vi "FollowPath.vi"(1 "Parameter String":string, 2 "Reinit":bool) -> (0 "Increment":bool)   [LabVIEW 2019]
uses:
  sensors.vi
  dsinstructions.vi
panel:
  out "Azimuth Goal Angle":dbl(knob) scale=180.0..-180.0
  out "FF Contribution":dbl
  out "Distance PID Tracking":cluster{"Goal Wheel Position":dbl, dbl}(graph)={"Goal Wheel Position"=0.0, -90.17571233858979}
  out "Distance Contribution Tracking":cluster{dbl, dbl, dbl}(graph)
  in  "N-Int Distance":i32=5 caption="N-Int"
  in  "N-Diff Distance":i32=10 caption="N-Diff"
  in  "Kd Distance":dbl=0.005
  in  "Ki Distance":dbl=0.2
  in  "Kp Distance":dbl=0.01
  out "Robot Position":cluster{dbl[], dbl[]}[](graph)
  in  "Plot":bool
  in  "N-Int Orientation":i32=10 caption="N-Int"
  in  "N-Diff Orientation":i32=10 caption="N-Diff"
  in  "Kd Orientation":dbl=0.0005
  in  "Ki Orientation":dbl
  in  "Kp Orientation":dbl=0.003
  out "Orientation PID Tracking":cluster{"Goal Wheel Position":dbl, dbl}(graph)={"Goal Wheel Position"=0.0, -90.17571233858979}
  out "Orientation Contribution Tracking":cluster{dbl, dbl, dbl}(graph)
  in  "Look-Ahead Time (s)":dbl=0.25
  in  "Search Window (s)":dbl=2.0
  # "Orientation Control"
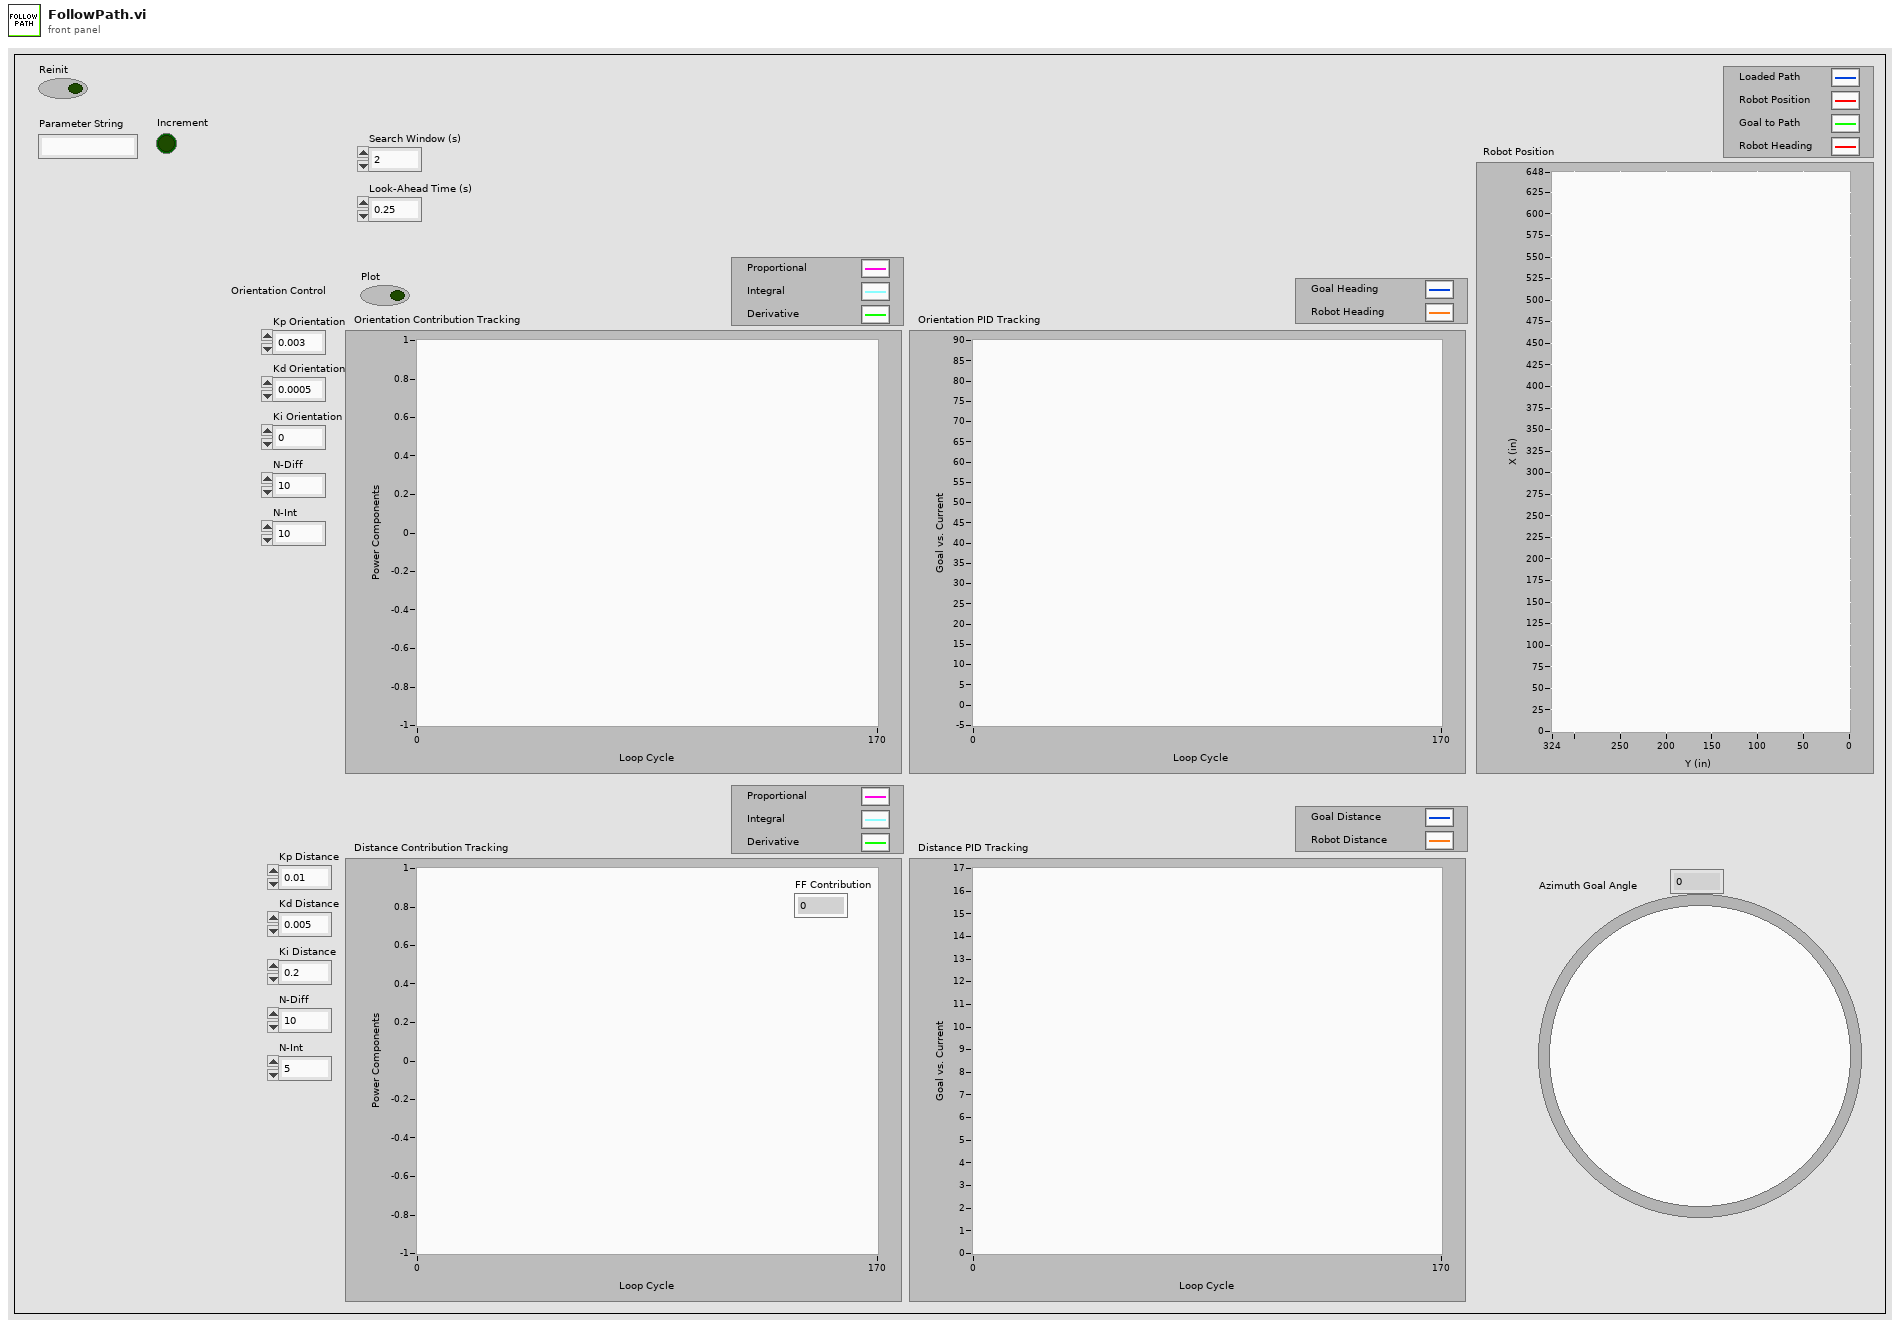
[diagram p1: front panel]
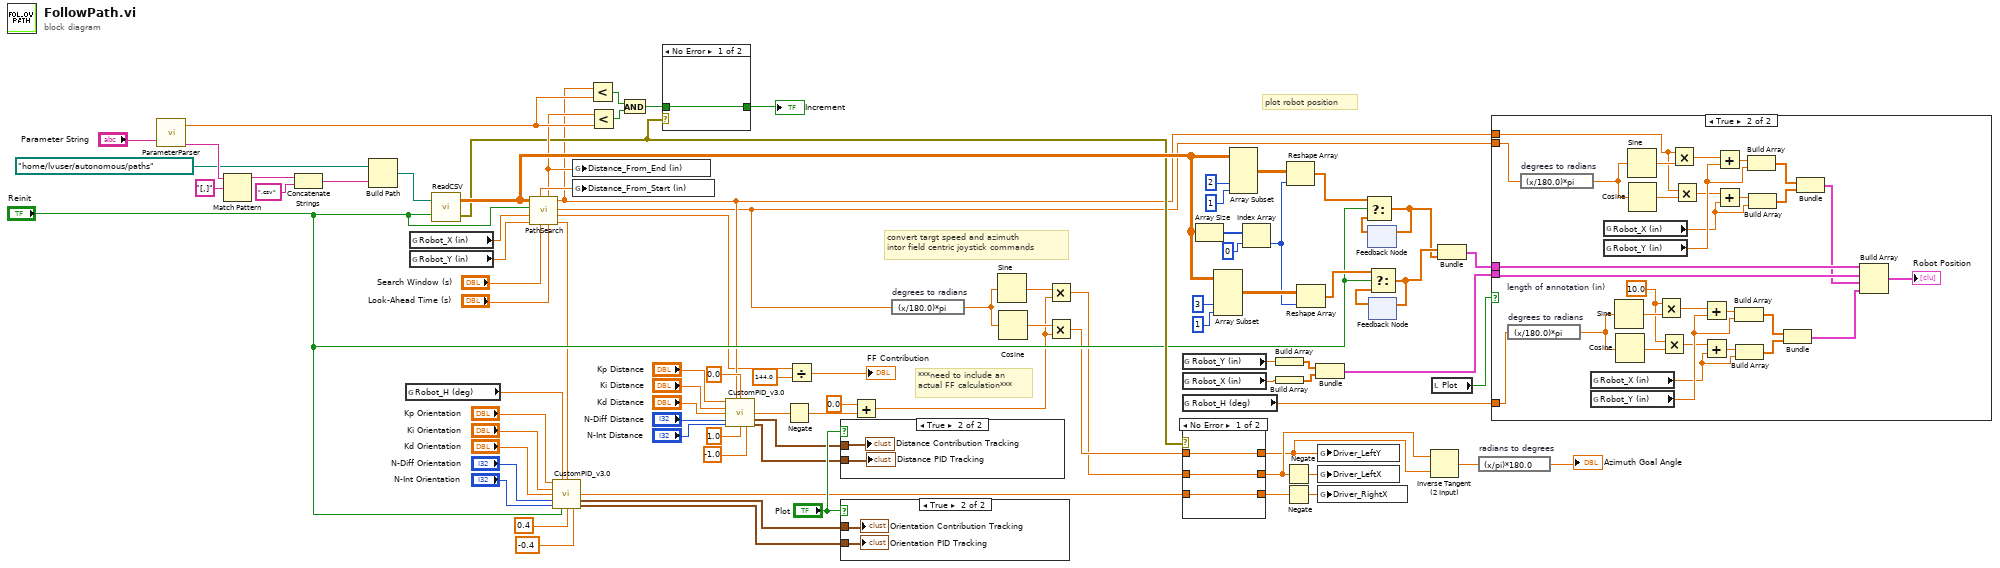
[diagram p0: block diagram]
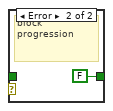
[diagram p3: hidden frame]
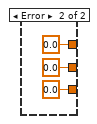
[diagram p4: hidden frame]
diagram:
  # "convert targt speed and azimuth\nintor field centric joystick commands"
  # "***need to include an \nactual FF calculation***"
  # "plot robot position"
  n1 = call "ParameterParser.vi"("Parameter String"="Parameter String") -> ("Remaining Parameter String"=w87:string, "Parameter"=w44:dbl)  [unwired: 1 in]
  n2 = Match Pattern(string=w87, regular expression="[,]") -> (before substring=w38:string)  [unwired: 1 in, 3 out]
  n3 = Concatenate Strings(w38, ".csv" ("string")) -> (w37:string)
  n4 = Build Path(base path=path "/home/lvuser/autonomous/paths" ("path"), name or relative path=w37) -> (appended path=w85:path)
  n5 = global read "sensors.vi" "Robot_H (deg)"() -> (w79:dbl)
  n6 = global read "sensors.vi" "Robot_X (in)"() -> (w83:dbl)
  n7 = global read "sensors.vi" "Robot_Y (in)"() -> (w82:dbl)
  n8 = call "ReadCSV.vi"("Reinit"="Reinit", "File Path (.csv)"=w85) -> ("File Open Eror"=w42:errorcluster, "Data (index by row)"=w57:dbl[][])
  n9 = call "PathSearch.vi"("Look-Ahead Time (s)"="Look-Ahead Time (s)", "Search Window (s)"="Search Window (s)", "Robot Y (in)"=w82, "Robot X (in)"=w83, "Reint"="Reinit", "Path"=w57) -> ("Angle Goal (deg)"=w1:dbl, "Velocity Goal (in/s)"=w21:dbl, "Angle To Goal (deg)"=w18:dbl, "Distance to Goal (in)"=w33:dbl, "Distance from End (in)"=w43:dbl, "Distance from Start (in)"=w84:dbl)
  n10 = call "CustomPID_v3.0.vi"("Kp"="Kp Orientation", "Process Variable"=w79, "Goal"=w1, "Ki"="Ki Orientation", "Kd"="Kd Orientation", "N-Diff"="N-Diff Orientation", "N-Int"="N-Int Orientation", "Reinit"="Reinit", "Max Ouput"=0.4, "Min Output"=-0.4) -> ("Command"=w15:dbl, "Contribution Tracking"=w78:cluster{dbl, dbl, dbl}, "PID Tracking"=w77:cluster{"Goal Wheel Position":dbl, dbl})  [unwired: 2 in, 1 out]
  n11 = global write "sensors.vi" "Distance_From_End (in)"(w43) -> ()
  n12 = global write "sensors.vi" "Distance_From_Start (in)"(w84) -> ()
  n13 = Less?(x=w33, y=w44) -> (x < y?=w59:bool)
  n14 = Less?(x=w43, y=w44) -> (x < y?=w58:bool)
  n15 = And(x=w59, y=w58) -> (x .and. y?=w41:bool)
  n16 = case shown="No Error" w42 {
    tunnel: [w90 FALSE] -> w40
    tunnel: w41 -> [w90 _]
    frame No Error {
    }
    frame Error {
      # "block progression"
    }
  }
  "Increment" <- w40
  n17 = call "CustomPID_v3.0.vi"("Kp"="Kp Distance", "Process Variable"=w33, "Goal"=0.0, "Ki"="Ki Distance", "Kd"="Kd Distance", "N-Diff"="N-Diff Distance", "N-Int"="N-Int Distance", "Max Ouput"=1.0, "Min Output"=-1.0) -> ("Command"=w22:dbl, "Contribution Tracking"=w24:cluster{dbl, dbl, dbl}, "PID Tracking"=w23:cluster{"Goal Wheel Position":dbl, dbl})  [unwired: 3 in, 1 out]
  n18 = Negate(x=w22) -> (-x=w4:dbl)
  n19 = Divide(x=w21, y=144.0) -> (x/y=→"FF Contribution":dbl)
  n20 = case shown="True" "Plot" {
    tunnel: w24 -> [_ w93]
    tunnel: w23 -> [_ w92]
    frame False {
    }
    frame True {
      "Distance Contribution Tracking" <- w93
      "Distance PID Tracking" <- w92
    }
  }
  n21 = case shown="True" "Plot" {
    tunnel: w78 -> [_ w95]
    tunnel: w77 -> [_ w94]
    frame False {
    }
    frame True {
      "Orientation Contribution Tracking" <- w95
      "Orientation PID Tracking" <- w94
    }
  }
  n22 = Add(x=0.0, y=w4) -> (x+y=w7:dbl)
  n23 = expression code="(x/180.0)*pi" "degrees to radians"(w18) -> (w10:dbl)
  n24 = Sine(x=w10) -> (sin(x)=w9:dbl)
  n25 = Cosine(x=w10) -> (cos(x)=w8:dbl)
  n26 = Multiply(x=w9, y=w7) -> (x*y=w5:dbl)
  n27 = Multiply(x=w8, y=w7) -> (x*y=w6:dbl)
  n28 = global read "sensors.vi" "Robot_Y (in)"() -> (w56:dbl)
  n29 = global read "sensors.vi" "Robot_X (in)"() -> (w55:dbl)
  n30 = global read "sensors.vi" "Robot_H (deg)"() -> (w39:dbl)
  n31 = case shown="No Error" w42 {
    tunnel: [w98 0.0] -> w14
    tunnel: w5 -> [w98 _]
    tunnel: [w96 0.0 ("upper limit")] -> w16
    tunnel: w6 -> [w97 _]
    tunnel: [w97 0.0] -> w13
    tunnel: w15 -> [w96 _]
    frame No Error {
    }
    frame Error {
    }
  }
  n32 = Array Size(array=w57) -> (size(s)=w62:i32[])
  n33 = Array Subset(array=w57, index (col)=3 ("index"), length (col)=1 ("length")) -> (w63:dbl[][])  [unwired: 2 in]
  n34 = Array Subset(array=w57, index (col)=2 ("index"), length (col)=1 ("length")) -> (w65:dbl[][])  [unwired: 2 in]
  n35 = Index Array(array=w62, index=0) -> (element=w60:i32)
  n36 = Build Array(w56) -> (w53:dbl[])
  n37 = Build Array(w55) -> (w54:dbl[])
  n38 = Negate(x=w14) -> (-x=w3:dbl)
  n39 = Negate(x=w16) -> (-x=w2:dbl)
  n40 = Reshape Array(w65, w60) -> (w46:dbl[])
  n41 = Reshape Array(w63, w60) -> (w64:dbl[])
  n42 = Bundle(w53, w54) -> (w48:cluster{dbl[], dbl[]})  [unwired: 1 in]
  n43 = global write "dsinstructions.vi" "Driver_LeftY"(w13) -> ()
  n44 = global write "dsinstructions.vi" "Driver_LeftX"(w3) -> ()
  n45 = global write "dsinstructions.vi" "Driver_RightX"(w2) -> ()
  n46 = feedback #1() -> (w50:dbl[])  [unwired: 1 in]
  n47 = Select(t=w46, s="Reinit", f=w50) -> (s? t:f=w51:dbl[])
  n48 = feedback-in #1(w51) -> ()
  n49 = feedback #2() -> (w49:dbl[])  [unwired: 1 in]
  n50 = Select(t=w64, s="Reinit", f=w49) -> (s? t:f=w52:dbl[])
  n51 = feedback-in #2(w52) -> ()
  n52 = Inverse Tangent (2 Input)(1:w13, 2:w14) -> (0:w11:dbl)
  n53 = local read "Plot"() -> (w45:bool)
  n54 = Bundle(w52, w51) -> (w47:cluster{dbl[], dbl[]})  [unwired: 1 in]
  n55 = expression code="(x/pi)*180.0" "radians to degrees"(w11) -> (→"Azimuth Goal Angle":dbl)
  n56 = case shown="True" w45 {
    tunnel: w48 -> [_ w131]
    tunnel: w47 -> [_ w130]
    tunnel: w33 -> [_ w118]
    tunnel: w18 -> [_ w117]
    tunnel: w39 -> [_ w104]
    frame False {
    }
    frame True {
      w103 = 10.0  # length of annotation (in)
      n57 = expression code="(x/180.0)*pi" "degrees to radians"(w104) -> (w105:dbl)
      n58 = expression code="(x/180.0)*pi" "degrees to radians"(w117) -> (w119:dbl)
      n59 = global read "sensors.vi" "Robot_X (in)"() -> (w114:dbl)
      n60 = global read "sensors.vi" "Robot_Y (in)"() -> (w115:dbl)
      n61 = global read "sensors.vi" "Robot_X (in)"() -> (w128:dbl)
      n62 = global read "sensors.vi" "Robot_Y (in)"() -> (w129:dbl)
      n63 = Sine(x=w105) -> (sin(x)=w106:dbl)
      n64 = Cosine(x=w105) -> (cos(x)=w107:dbl)
      n65 = Sine(x=w119) -> (sin(x)=w120:dbl)
      n66 = Cosine(x=w119) -> (cos(x)=w121:dbl)
      n67 = Multiply(x=w103, y=w106) -> (x*y=w108:dbl)
      n68 = Multiply(x=w103, y=w107) -> (x*y=w109:dbl)
      n69 = Multiply(x=w118, y=w120) -> (x*y=w122:dbl)
      n70 = Multiply(x=w118, y=w121) -> (x*y=w123:dbl)
      n71 = Add(x=w108, y=w115) -> (x+y=w110:dbl)
      n72 = Add(x=w109, y=w114) -> (x+y=w111:dbl)
      n73 = Add(x=w122, y=w129) -> (x+y=w124:dbl)
      n74 = Add(x=w123, y=w128) -> (x+y=w125:dbl)
      n75 = Build Array(w110, w115) -> (w112:dbl[])
      n76 = Build Array(w111, w114) -> (w113:dbl[])
      n77 = Build Array(w124, w129) -> (w126:dbl[])
      n78 = Build Array(w125, w128) -> (w127:dbl[])
      n79 = Bundle(w112, w113) -> (w102:cluster{dbl[], dbl[]})  [unwired: 1 in]
      n80 = Bundle(w126, w127) -> (w116:cluster{dbl[], dbl[]})  [unwired: 1 in]
      n81 = Build Array(w130, w131, w116, w102) -> (→"Robot Position":cluster{dbl[], dbl[]}[])
    }
  }
